vi "C4Ftr_getSelectedList.vi"(0 "c4Ftr in":refnum<k24>, 11 "error in":errorcluster) -> (4 "c4Ftr out":refnum<k24>, 6 "selector list out":string[](array[string]), 15 "error out":errorcluster)   [LabVIEW 2015, in "libC4HdlLV.lvlib"]
uses:
  libC4HdlLV.lvlib
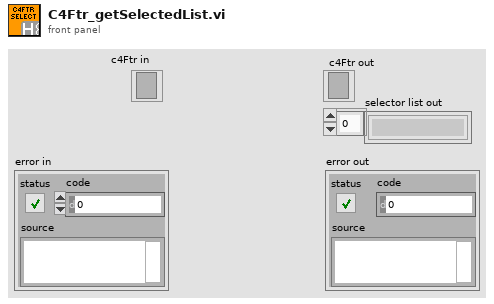
[diagram p1: front panel]
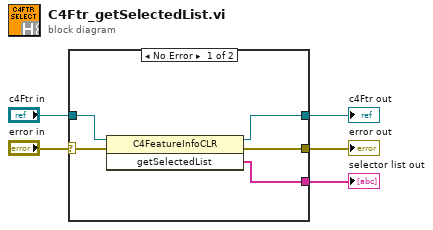
[diagram p0: block diagram]
diagram:
  n1 = case shown="No Error" "error in" {
    selector: "error in" -> [w10 w11]
    tunnel: "c4Ftr in" -> [w9 w12]
    tunnel: [w8 w11] -> w3
    tunnel: [w7 w12] -> w2
    tunnel: [w6 _] -> w1
    frame No Error {
      n2 = invoke class="C4FeatureInfoCLR" method="getSelectedList"(reference=w9, error in=w10) -> (reference out=w7:refnum<k24>, error out=w8:errorcluster, "getSelectedList"=w6:string[])  [unwired: 1 in]
    }
    frame Error {
    }
  }
  "error out" <- w3
  "c4Ftr out" <- w2
  "selector list out" <- w1
